vi "Unreserve Callback.vi"(8 "error in (no error)":errorcluster, 10 "session reservation":refnum<class "Session Reservation.lvclass">, 11 "reservation observer in":refnum<class "Reservation Observer.lvclass">) -> (0 "error out":errorcluster, 3 "reservation observer out":refnum<class "Reservation Observer.lvclass">)   [LabVIEW 2020, in "MeasurementLink Measurement Server.lvlib" / "Reservation Observer.lvclass"]
uses:
  Reservation Observer.lvclass
  MeasurementLink Session Management/Session Reservation/Session Reservation.lvclass
  Reservation Observer.lvclass/Reservation Observer.ctl
  Classes/MeasurementContext/MeasurementContext.lvclass
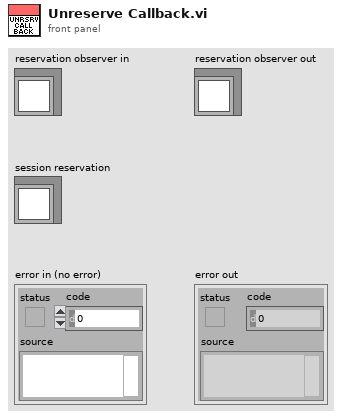
[diagram p1: front panel]
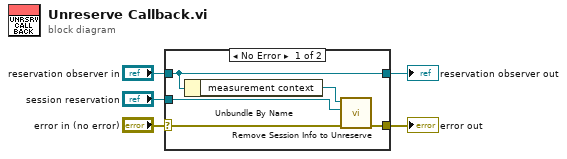
[diagram p0: block diagram]
diagram:
  n1 = case shown="No Error" "error in (no error)" {
    selector: "error in (no error)" -> [w7 w11]
    tunnel: [w10 w12] -> w4
    tunnel: "reservation observer in" -> [w10 w12]
    tunnel: [w6 w11] -> w2
    tunnel: "session reservation" -> [w8 _]
    frame No Error {
      n2 = Unbundle By Name(w10) -> ("measurement context"=w9:refnum<class "MeasurementContext.lvclass">)
      n3 = call "Remove Session Info to Unreserve.vi"("error in"=w7, "session reservation"=w8, "measurement context in"=w9) -> ("error out"=w6:errorcluster)  [unwired: 7 in, 1 out]
    }
    frame Error {
    }
  }
  "error out" <- w2
  "reservation observer out" <- w4
